vi "Launcher.vi"() -> ()   [LabVIEW 2020]
uses:
  Actors/First Actor/First Actor/First Actor.lvclass
  C:/Program Files (x86)/National Instruments/LabVIEW 2020/vi.lib/ActorFramework/Actor/Actor.lvclass
  Actors/First Actor/First Actor Messages/ShowMSG Msg/ShowMSG Msg.lvclass/ShowMSG Msg.ctl
  <vilib>/ActorFramework/Message Enqueuer/Message Enqueuer.lvclass/Message Enqueuer.ctl
  <vilib>/ActorFramework/Message Enqueuer/Enqueue.vi
  Actors/First Actor/First Actor Messages/ShowMSG Msg/ShowMSG Msg.lvclass
  C:/Program Files (x86)/National Instruments/LabVIEW 2020/vi.lib/ActorFramework/Message/Message.lvclass
  <vilib>/ActorFramework/Stop Msg/Stop Msg.lvclass
  <vilib>/ActorFramework/Message Priority Queue/Priority Enqueue.vi
  <vilib>/ActorFramework/Actor/Actor.lvclass
panel:
  in  "Open Actor Core front panel? (F)":bool
  in  "MSG to Display":string
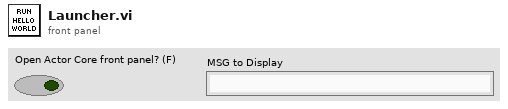
[diagram p1: front panel]
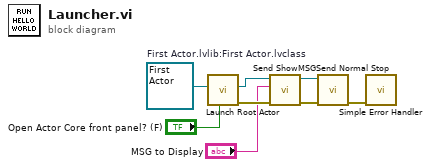
[diagram p0: block diagram]
diagram:
  w8 = refnum<class "First Actor.lvclass"> refnum  # First Actor.lvlib:First Actor.lvclass
  n1 = call <vilib>:"Launch Root Actor.vi"("Open Actor Core front panel? (F)"="Open Actor Core front panel? (F)", "Actor"=w8) -> ("error out"=w6:errorcluster, "Actor's Enqueuer"=w7:refnum<class "Message Enqueuer.lvclass">)  [unwired: 8 in]
  n2 = call "Send ShowMSG.vi"("error in (no error)"=w6, "String"="MSG to Display", "Message Enqueuer"=w7) -> ("error out"=w4:errorcluster, "Message Enqueuer out"=w3:refnum<class "Message Enqueuer.lvclass">)  [unwired: 7 in]
  n3 = call <vilib>:"Send Normal Stop.vi"("error in (no error)"=w4, "Message Enqueuer"=w3) -> ("error out"=w2:errorcluster)  [unwired: 9 in]
  n4 = call <vilib>:"Simple Error Handler.vi"("error in (no error)"=w2) -> ()  [unwired: 4 in, 5 out]
